vi "connect.vi"(8 "error in":errorcluster, 11 "deviceAddress":string="10.99.70.243") -> (0 "error out":errorcluster, 3 "deviceHandle":i32)   [LabVIEW 2016]
uses:
  DLLHandler/Release/LabVIEWJSON.dll
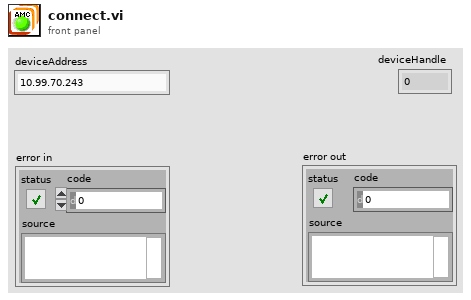
[diagram p1: front panel]
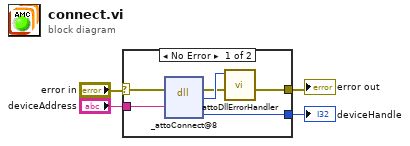
[diagram p0: block diagram]
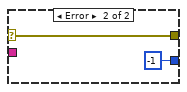
[diagram p2: hidden frame]
diagram:
  n1 = case shown="No Error" "error in" {
    selector: "error in" -> [w5 w12]
    tunnel: "deviceAddress" -> [w10 _]
    tunnel: [w9 -1 ("deviceHandle")] -> w2
    tunnel: [w6 w12] -> w1
    frame No Error {
      n2 = dll-call lib="C:/Users/schieda/OneDrive - WITTENSTEIN SE/Desktop/LabVIEW/API_Autogen_v1.3_DSc/generatedAPIs/AMC_VIs_DLL (for older LV Versions only)/DLLHandler/Release/LabVIEWJSON.dll" fn="_attoConnect@8"(error in=w5, "deviceAddress"=w10) -> (error out=w7:errorcluster, "rc"=w8:i32, "deviceHandle"=w9:i32)  [unwired: 4 in, 1 out]
      n3 = call "attoDllErrorHandler.vi"("error in"=w7, "rc"=w8) -> ("error out"=w6:errorcluster)  [unwired: 9 in]
    }
    frame Error {
    }
  }
  "deviceHandle" <- w2
  "error out" <- w1
